vi "Matrix RMS.vi"(8 "Original Matrix":dbl[][](array[numeric]) format="%0.3f", 9 "Iterative Matrix":dbl[][](array[numeric]), 11 "error in (no error)":errorcluster) -> (0 "RMS":dbl, 3 "error out":errorcluster)   [LabVIEW 2012, in "LightPipes.lvlib"]
uses:
  LightPipes.lvlib
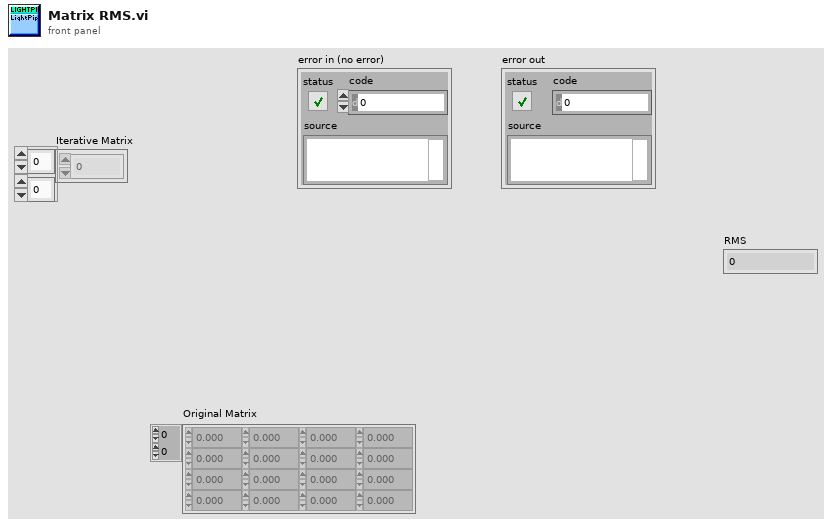
[diagram p1: front panel]
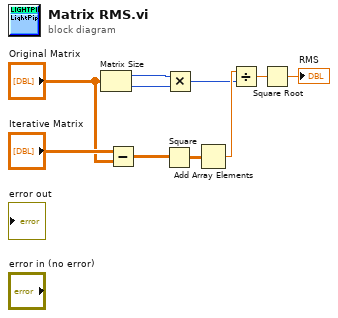
[diagram p0: block diagram]
diagram:
  n1 = Matrix Size(0:"Original Matrix") -> (1:w4:i32, 2:w3:i32)
  n2 = Subtract(x="Iterative Matrix", y="Original Matrix") -> (x-y=w10:dbl[][])
  n3 = Square(x=w10) -> (x^2=w9:dbl[][])
  n4 = Multiply(x=w4, y=w3) -> (x*y=w1:i32)
  n5 = Add Array Elements(numeric array=w9) -> (sum=w7:dbl)
  n6 = Divide(x=w7, y=w1) -> (x/y=w6:dbl)
  n7 = Square Root(x=w6) -> (sqrt(x)=→"RMS":dbl)
